vi "Read ELAN Master.vi"(8 "error in (no error)":errorcluster, 11 "ELAN in":refnum<class "ELAN.lvclass">) -> (0 "error out":errorcluster, 2 "Network Master":refnum<class "ELAN Master.lvclass">, 3 "ELAN out":refnum<class "ELAN.lvclass">)   [LabVIEW 2021, in "ELAN.lvclass"]
uses:
  ELAN.lvclass
  D:/my_projects/projects/Algorithms/Labview/21/Master CR/Master CR.lvclass
  Network Protocol/ELAN Master/ELAN Master.lvclass
  Master CR.lvclass/Master CR.ctl
  Master CR.lvclass
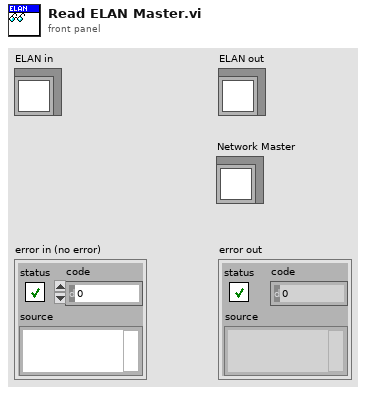
[diagram p1: front panel]
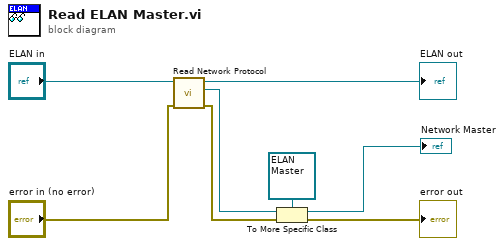
[diagram p0: block diagram]
diagram:
  n1 = call "Read Network Protocol.vi"("error in (no error)"="error in (no error)", "Master CR in"="ELAN in") -> ("error out"=w5:errorcluster, "Network Protocol"=w2:refnum<class "Network Protocol.lvclass">, "Master CR out"=→"ELAN out":refnum<class "ELAN.lvclass">)  [unwired: 7 in]
  n2 = To More Specific Class(target class=refnum<class "ELAN Master.lvclass"> refnum ("Network Master"), reference=w2, error in=w5) -> (specific class reference=→"Network Master":refnum<class "ELAN Master.lvclass">, error out=→"error out":errorcluster)
